vi "3.9.2-Low Pass.vi"(1 "Signal In":dbl, 2 "Gain":dbl) -> (0 "Signal Out":dbl)   [LabVIEW 2010]
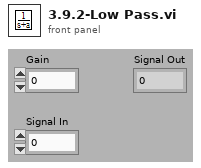
[diagram p1: front panel]
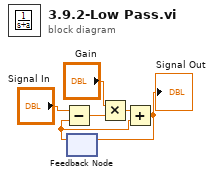
[diagram p0: block diagram]
diagram:
  n1 = feedback #1() -> (w4:dbl)  [unwired: 1 in]
  n2 = Subtract(x="Signal In", y=w4) -> (x-y=w2:dbl)
  n3 = Multiply(x="Gain", y=w2) -> (x*y=w3:dbl)
  n4 = Add(x=w3, y=w4) -> (x+y=w6:dbl)
  "Signal Out" <- w6
  n5 = feedback-in #1(w6) -> ()
